vi "APTmotorOpen.vi"(4 "error in (no error)":errorcluster) -> (0 "error out":errorcluster, 3 "reference out":refnum<k7>[](array[refnum]))   [LabVIEW 2015]
panel:
  in  "APTPZMotor x":refnum<k7>(container)
  in  "APTPZMotor y":refnum<k7>(container)
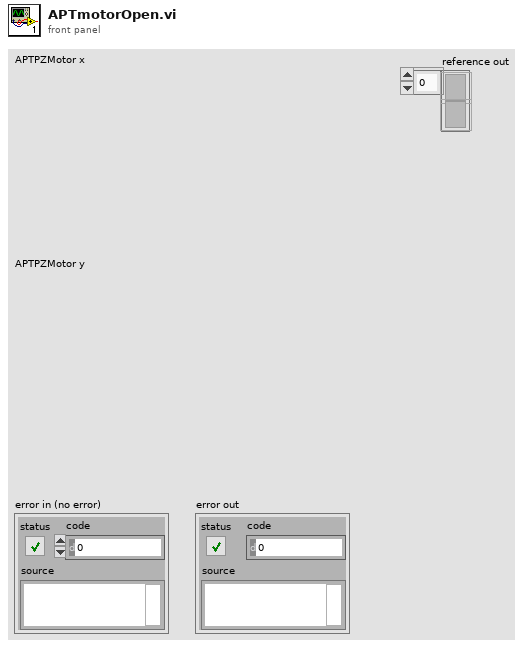
[diagram p1: front panel]
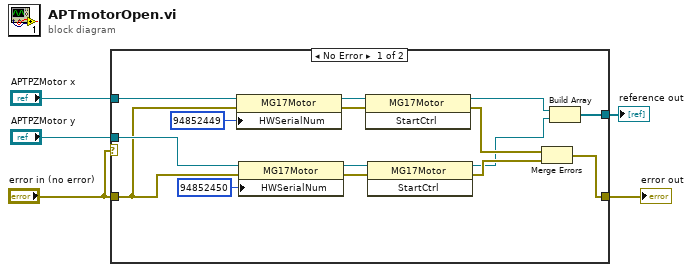
[diagram p0: block diagram]
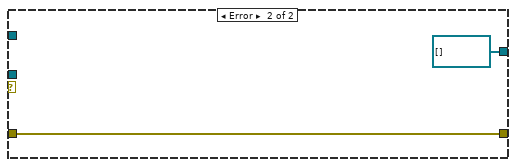
[diagram p2: hidden frame]
diagram:
  n1 = case shown="No Error" "error in (no error)" {
    tunnel: "APTPZMotor y" -> [w20 _]
    tunnel: "error in (no error)" -> [w13 w22]
    tunnel: [w9 w22] -> w4
    tunnel: "APTPZMotor x" -> [w16 _]
    tunnel: [w7 refnum<k7>[] []] -> w1
    frame No Error {
      n2 = property class="MG17Motor"(reference=w16, error in=w13, "HWSerialNum"=94852449) -> (reference out=w15:refnum<k7>, error out=w14:errorcluster)
      n3 = property class="MG17Motor"(reference=w20, error in=w13, "HWSerialNum"=94852450) -> (reference out=w18:refnum<k7>, error out=w17:errorcluster)
      n4 = invoke class="MG17Motor" method="StartCtrl"(reference=w15, error in=w14) -> (reference out=w6:refnum<k7>, error out=w10:errorcluster)  [unwired: 1 in, 1 out]
      n5 = invoke class="MG17Motor" method="StartCtrl"(reference=w18, error in=w17) -> (reference out=w8:refnum<k7>, error out=w11:errorcluster)  [unwired: 1 in, 1 out]
      n6 = Merge Errors(w10, w11) -> (w9:errorcluster)
      n7 = Build Array(w6, w8) -> (w7:refnum<k7>[])
    }
    frame Error {
    }
  }
  "error out" <- w4
  "reference out" <- w1
